vi "Angle-Coordinate Points.vi"(10 "radius":dbl, 11 "theta":dbl) -> (3 "x,y coords":cluster{dbl, dbl})   [LabVIEW 2019]
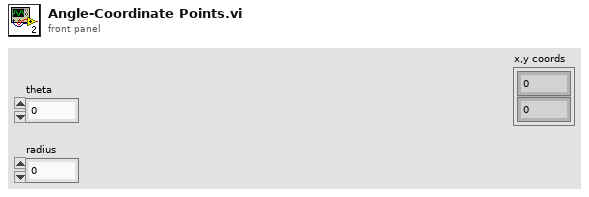
[diagram p1: front panel]
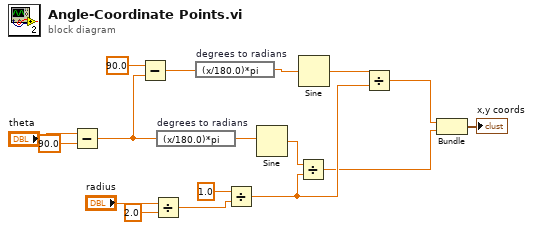
[diagram p0: block diagram]
diagram:
  n1 = Subtract(x="theta", y=90.0) -> (x-y=w4:dbl)
  n2 = Subtract(x=90.0, y=w4) -> (x-y=w9:dbl)
  n3 = Divide(x="radius", y=2.0) -> (x/y=w1:dbl)
  n4 = expression code="(x/180.0)*pi" "degrees to radians"(w4) -> (w7:dbl)
  n5 = expression code="(x/180.0)*pi" "degrees to radians"(w9) -> (w8:dbl)
  n6 = Divide(x=1.0, y=w1) -> (x/y=w13:dbl)
  n7 = Sine(x=w7) -> (sin(x)=w17:dbl)
  n8 = Divide(x=w17, y=w13) -> (x/y=w11:dbl)
  n9 = Sine(x=w8) -> (sin(x)=w14:dbl)
  n10 = Divide(x=w14, y=w13) -> (x/y=w12:dbl)
  n11 = Bundle(w12, w11) -> (→"x,y coords":cluster{dbl, dbl})  [unwired: 1 in]
